vi "RD Digital IO Input Status.vi"(8 "error in (no error)":errorcluster caption="错误输入（无错误）", 10 "reads":u32, 11 "handle":u32) -> (0 "error out":errorcluster caption="错误输出", 1 "function return":i32, 2 "reads out":u32, 3 "handle out":u32)   [LabVIEW 2018, in "InstrumentsPlayground.lvlib"]
doc: "CLIFFAPI int CliffDigitalIOInputStatus(FT_HANDLE handle,uint* reads);"
uses:
  InstrumentsPlayground.lvlib
  LabVIEW lib/InstrumentsPlayground.dll
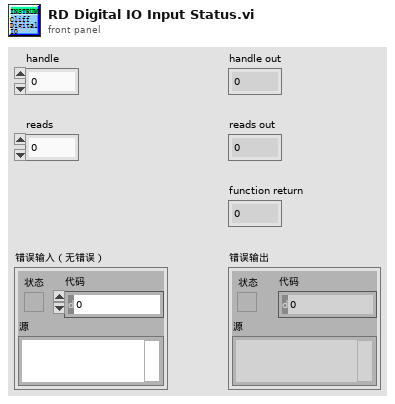
[diagram p1: front panel]
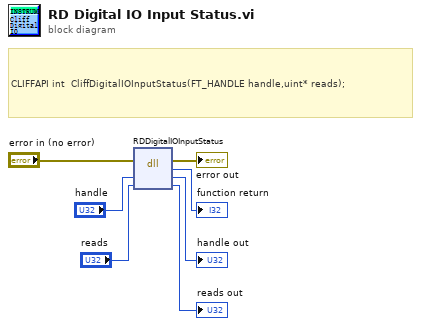
[diagram p0: block diagram]
diagram:
  # "CLIFFAPI int  CliffDigitalIOInputStatus(FT_HANDLE handle,uint* reads);"
  n1 = dll-call lib="E:/work/YZCourse_Xtext/Cliff/API/LabVIEW lib/InstrumentsPlayground.*" fn="RDDigitalIOInputStatus"(error in="error in (no error)", "handle"="handle", "reads"="reads") -> (error out=→"error out":errorcluster, "返回类型"=→"function return":i32, "handle"=→"handle out":u64, "reads"=→"reads out":u32)  [unwired: 2 in, 1 out]
